vi "FRCts20_WebMethods_ESP_RequestArray.vi"(8 "error in (no error)":errorcluster, 9 "Requests":T3, 10 "Return Type":T4="mobile", 11 "httpRequestID":u32) -> (0 "error out":errorcluster, 3 "httpRequestID out":u32)   [LabVIEW 2014, in "FRCts20_WebMethods.lvlib"]
uses:
  FRCts20_WebMethods.lvlib
  Controls/FRCts20_WebMethods_ctl_returntype.ctl
  Controls/FRCts20_WebMethods_ctl_requestarray.ctl
  Backend/source/VI Source/FRCts20_Backend_API/FRCts20_Backend_API_Status.ctl
  Backend/source/VI Source/FRCts20_Backend_API/FRCts20_Backend_API_SW.ctl
  Controls/FRCts20_WebMethods_Globals.vi
  <vilib>/wsapi/subVIs/Set String ESP Variable.vi
  <vilib>/wsapi/subVIs/Set Integer ESP Variable.vi
  Backend/source/VI Source/FRCts20_Backend_API/FRCts20_Backend_API.lvlib
  <vilib>/wsapi/NI_WebServices.lvlib
  Backend/source/VI Source/FRCts20_Backend_API/FRCts20_Backend_API_Command_Competition.ctl
  Backend/source/VI Source/FRCts20_Backend_API/FRCts20_Backend_API_Competition.ctl
  Backend/source/VI Source/INI_Accessor/FRCts20_Backend_INI Controller.lvclass
  Backend/source/VI Source/FRCts20_Backend_API/FRCts20_Backend_API_Event.vi
  Backend/source/VI Source/FRCts20_Backend_API/FRCts20_Backend_API_Event.ctl
panel:
  in  "Status (hidden)":T1
  in  "SWType (hidden)":T2
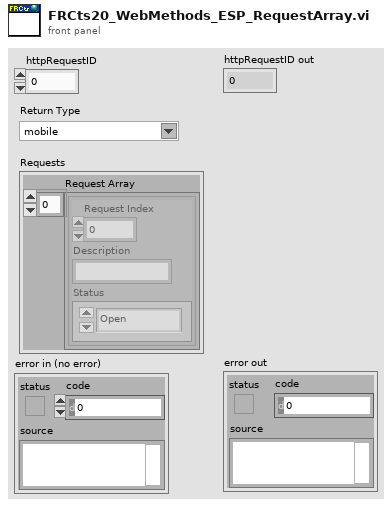
[diagram p1: front panel]
types:
  T1 = typedef "FRCts20_Backend_API.lvlib/FRCts20_Backend_API_Status.ctl" = enum16{"Open", "In Work", "Closed"}
  T2 = typedef "FRCts20_Backend_API.lvlib/FRCts20_Backend_API_SW.ctl" = string
  T3 = typedef "FRCts20_WebMethods.lvlib/FRCts20_WebMethods_ctl_requestarray.ctl" = cluster{"Request Array":cluster{"Request Index":u32, "Description":string, "Status":T1}[]}
  T4 = typedef "FRCts20_WebMethods.lvlib/FRCts20_WebMethods_ctl_returntype.ctl" = string
  T5 = typedef "FRCts20_Backend_API.lvlib/FRCts20_Backend_API_Event.ctl" = cluster{"Event Index":u32, "Name":string, "Start Time":timestamp, "End Time":timestamp, "Teams":cluster{"Team Index":u32, "Team Number":u32, "Requests":cluster{"Request Number":u32, "Description":string}[], "Has Open Issue":bool}[], "SWType":T2, "APIReturn":string}
  T6 = typedef "FRCts20_Backend_API.lvlib/FRCts20_Backend_API_Competition.ctl" = cluster{"Name":string, "Start Date":timestamp, "Duration":u8, "Divisions":string[], "APIReturn":string}
  T7 = typedef "FRCts20_Backend_API.lvlib/FRCts20_Backend_API_Command_Competition.ctl" = string
  T8 = cluster{"Request Index":u32, "Description":string, "Status":T1}[]
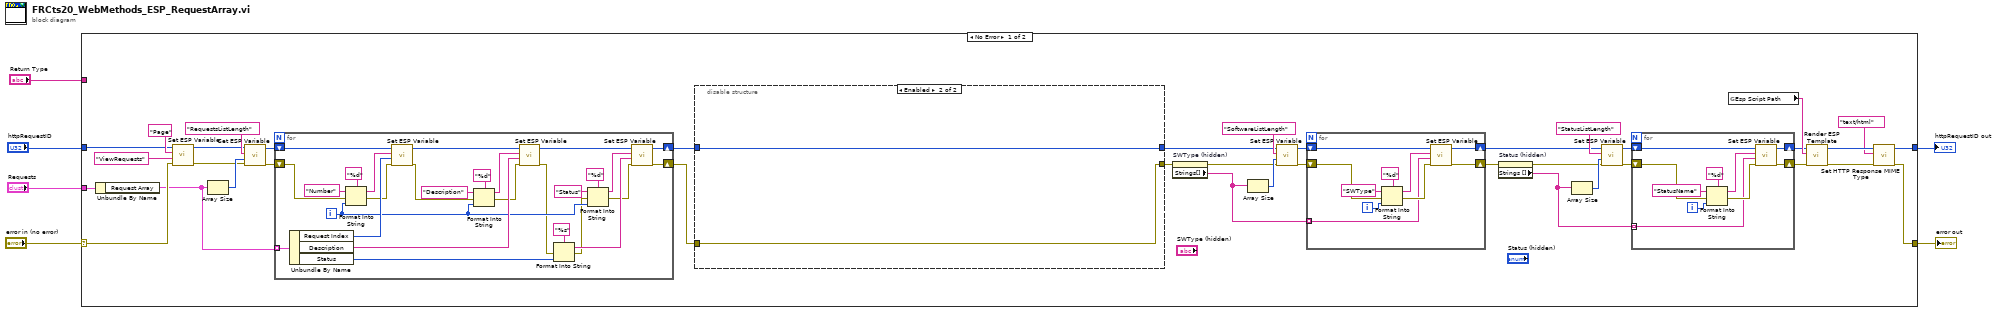
[diagram p0: block diagram]
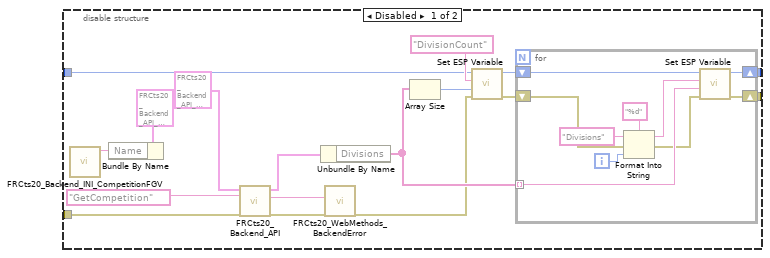
[diagram p2: hidden frame]
diagram:
  n1 = case shown="No Error" "error in (no error)" {
    selector: "error in (no error)" -> [w28 w123]
    tunnel: "httpRequestID" -> [w31 w122]
    tunnel: [w42 w122] -> w3
    tunnel: [w41 w123] -> w2
    tunnel: "Return Type" -> [_ _]
    tunnel: "Requests" -> [w34 _]
    frame No Error {
      n2 = Unbundle By Name(w34) -> ("Request Array"=w27:T8)
      n3 = call-poly <vilib>:"Set ESP Variable.vi"("error in (no error)"=w28, "value"="ViewRequests", "key"="Page", "httpRequestID"=w31) -> ("error out"=w30:errorcluster, "httpRequestID out"=w29:u32)  [unwired: 6 in]
      n4 = Array Size(array=w27) -> (size(s)=w38:i32)
      n5 = call-poly <vilib>:"Set ESP Variable.vi"("error in (no error)"=w30, "value"=w38, "key"="RequestsListLength", "httpRequestID"=w29) -> ("error out"=w36:errorcluster, "httpRequestID out"=w35:u32)  [unwired: 6 in]
      n6 = for {
        shift-right: [w106] -> w25
        shift-left: w36 -> [w100]
        shift-right: [w105] -> w26
        shift-left: w35 -> [w121]
        tunnel: w27 -> [w117] mode=indexing
        i -> [w107]
        n7 = Unbundle By Name(w117) -> ("Request Index"=w116:u32, "Description"=w111:string, "Status"=w103:T1)
        n8 = Format Into String(format string="%d", initial string="Number", error in=w100, w107) -> (resulting string=w119:string, error out=w99:errorcluster)
        n9 = call-poly <vilib>:"Set ESP Variable.vi"("error in (no error)"=w99, "value"=w116, "key"=w119, "httpRequestID"=w121) -> ("error out"=w98:errorcluster, "httpRequestID out"=w114:u32)  [unwired: 6 in]
        n10 = Format Into String(format string="%d", initial string="Description", error in=w98, w107) -> (resulting string=w110:string, error out=w97:errorcluster)
        n11 = call-poly <vilib>:"Set ESP Variable.vi"("error in (no error)"=w97, "value"=w111, "key"=w110, "httpRequestID"=w114) -> ("error out"=w96:errorcluster, "httpRequestID out"=w115:u32)  [unwired: 6 in]
        n12 = Format Into String(format string="%s", error in=w96, w103) -> (resulting string=w101:string, error out=w95:errorcluster)  [unwired: 1 in]
        n13 = Format Into String(format string="%d", initial string="Status", error in=w95, w107) -> (resulting string=w104:string, error out=w94:errorcluster)
        n14 = call-poly <vilib>:"Set ESP Variable.vi"("error in (no error)"=w94, "value"=w101, "key"=w104, "httpRequestID"=w115) -> ("error out"=w106:errorcluster, "httpRequestID out"=w105:u32)  [unwired: 6 in]
      }
      n15 = disable-structure shown="Enabled" {
        disable-tunnel: w26 -> [w54 w73]
        disable-tunnel: w25 -> [w53 w72]
        disable-tunnel: [w49 w73] -> w21
        disable-tunnel: [w48 w72] -> w12
        frame Disabled {
          n16 = call "FRCts20_Backend_INI_CompetitionFGV.vi"() -> ("Value out"=w46:string)  [unwired: 11 in]
          n17 = Bundle By Name(cluster=T6 {"Name"="", "Start Date"=timestamp(0 s since 1904-01-01), "Duration"=0, "Divisions"=[], "APIReturn"=""} ("Competition In"), "Name"=w46) -> ()  [unwired: 1 out]
          n18 = call-poly "FRCts20_Backend_API.vi"("error in (no error)"=w53, "Command"=T7 "GetCompetition", "Event In"=T5 {"Event Index"=0, "Name"="", "Start Time"=timestamp(0 s since 1904-01-01), "End Time"=timestamp(0 s since 1904-01-01), "Teams"=[], "SWType"="", "APIReturn"=""}) -> ("error out"=w52:errorcluster, "Status"=w51:string, "Event Out"=w61:T5)  [unwired: 6 in]
          n19 = Unbundle By Name(w61) -> ("Divisions"=w58:string[])
          n20 = call "FRCts20_WebMethods_BackendError.vi"("error in (no error)"=w52, "Status"=w51) -> ("error out"=w50:errorcluster)  [unwired: 8 in, 1 out]
          n21 = Array Size(array=w58) -> (size(s)=w60:i32)
          n22 = call-poly <vilib>:"Set ESP Variable.vi"("error in (no error)"=w50, "value"=w60, "key"="DivisionCount", "httpRequestID"=w54) -> ("error out"=w57:errorcluster, "httpRequestID out"=w56:u32)  [unwired: 6 in]
          n23 = for {
            tunnel: w58 -> [w66] mode=indexing
            shift-right: [w71] -> w48
            shift-left: w57 -> [w63]
            shift-right: [w64] -> w49
            shift-left: w56 -> [w70]
            i -> [w68]
            n24 = Format Into String(format string="%d", initial string="Divisions", error in=w63, w68) -> (resulting string=w67:string, error out=w62:errorcluster)
            n25 = call-poly <vilib>:"Set ESP Variable.vi"("error in (no error)"=w62, "value"=w66, "key"=w67, "httpRequestID"=w70) -> ("error out"=w71:errorcluster, "httpRequestID out"=w64:u32)  [unwired: 6 in]
          }
        }
        frame Enabled {
        }
      }
      n26 = property on="SWType (hidden)" class="CmbBox (strict)"(error in=w12) -> (error out=w11:errorcluster, "Strings[]"=w19:string[])  [unwired: 1 in, 1 out]
      n27 = Array Size(array=w19) -> (size(s)=w20:i32)
      n28 = call-poly <vilib>:"Set ESP Variable.vi"("error in (no error)"=w11, "value"=w20, "key"="SoftwareListLength", "httpRequestID"=w21) -> ("error out"=w23:errorcluster, "httpRequestID out"=w24:u32)  [unwired: 6 in]
      n29 = for {
        shift-right: [w93] -> w10
        shift-left: w23 -> [w86]
        shift-right: [w87] -> w15
        shift-left: w24 -> [w92]
        tunnel: w19 -> [w84] mode=indexing
        i -> [w90]
        n30 = Format Into String(format string="%d", initial string="SWType", error in=w86, w90) -> (resulting string=w89:string, error out=w85:errorcluster)
        n31 = call-poly <vilib>:"Set ESP Variable.vi"("error in (no error)"=w85, "value"=w84, "key"=w89, "httpRequestID"=w92) -> ("error out"=w93:errorcluster, "httpRequestID out"=w87:u32)  [unwired: 6 in]
      }
      n32 = property on="Status (hidden)" class="Enum (strict)"(error in=w10) -> (error out=w7:errorcluster, "Strings []"=w8:string[])  [unwired: 1 in, 1 out]
      n33 = Array Size(array=w8) -> (size(s)=w9:i32)
      n34 = call-poly <vilib>:"Set ESP Variable.vi"("error in (no error)"=w7, "value"=w9, "key"="StatusListLength", "httpRequestID"=w15) -> ("error out"=w17:errorcluster, "httpRequestID out"=w16:u32)  [unwired: 6 in]
      n35 = for {
        shift-right: [w83] -> w14
        shift-left: w17 -> [w76]
        shift-right: [w77] -> w13
        shift-left: w16 -> [w82]
        tunnel: w8 -> [w74] mode=indexing
        i -> [w80]
        n36 = Format Into String(format string="%d", initial string="StatusName", error in=w76, w80) -> (resulting string=w79:string, error out=w75:errorcluster)
        n37 = call-poly <vilib>:"Set ESP Variable.vi"("error in (no error)"=w75, "value"=w74, "key"=w79, "httpRequestID"=w82) -> ("error out"=w83:errorcluster, "httpRequestID out"=w77:u32)  [unwired: 6 in]
      }
      n38 = global read "FRCts20_WebMethods_Globals.vi" "Esp Script Path"() -> (w40:string)
      n39 = call <vilib>:"Render ESP Template.vi"("error in (no error)"=w14, "espName"=w40, "httpRequestID"=w13) -> ("error out"=w43:errorcluster, "httpRequestID out"=w44:u32)  [unwired: 7 in]
      n40 = call <vilib>:"Set HTTP Response MIME Type.vi"("error in (no error)"=w43, "MIME type (text/html)"="text/html", "httpRequestID"=w44) -> ("error out"=w41:errorcluster, "httpRequestID out"=w42:u32)  [unwired: 7 in]
    }
    frame Error {
    }
  }
  "httpRequestID out" <- w3
  "error out" <- w2
